vi "PQsetNoticeProcessor.vi"(8 "error in (no error)":errorcluster, 9 "arg":u32) -> (0 "error out":errorcluster, 1 "PQnoticeReceiver":u32, 2 "arg out":u32)   [LabVIEW 2019, in "libpqlv.lvlib"]
uses:
  libpqlv.lvlib
  libpq.dll
panel:
  in  "proc":u32
  in  "conn":u32
  out "conn_out":u32
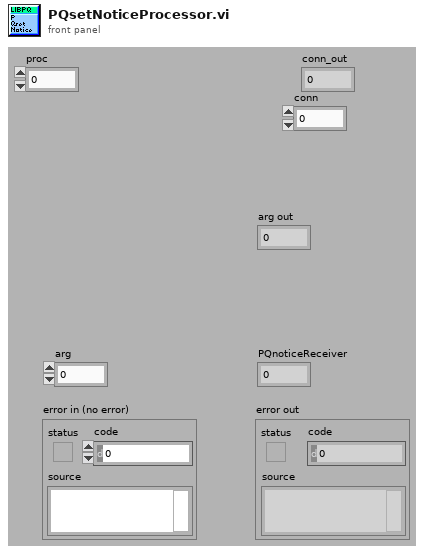
[diagram p1: front panel]
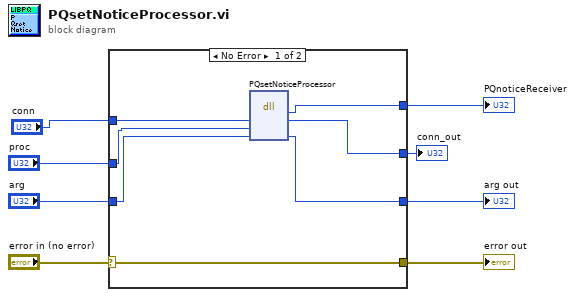
[diagram p0: block diagram]
diagram:
  n1 = case shown="No Error" "error in (no error)" {
    selector: "error in (no error)" -> [w15 w18]
    tunnel: [w15 w18] -> w7
    tunnel: [w14 _] -> w6
    tunnel: [w13 w16] -> w3
    tunnel: "arg" -> [w12 w17]
    tunnel: [w11 w17] -> w4
    tunnel: "conn" -> [w10 w16]
    tunnel: "proc" -> [w9 _]
    frame No Error {
      n2 = dll-call lib="libpq.*" fn="PQsetNoticeProcessor"("conn"=w10, "proc"=w9, "arg"=w12) -> ("PQnoticeReceiver"=w14:u32, "conn"=w13:u32, "arg"=w11:u32)  [unwired: 4 in, 2 out]
    }
    frame Error {
    }
  }
  "PQnoticeReceiver" <- w6
  "arg out" <- w4
  "error out" <- w7
  "conn_out" <- w3
